vi "Modbus Close.vi"(8 "error in (no error)":errorcluster, 11 "VISA resource in":refnum<visa-resource-name>) -> (0 "error out":errorcluster)   [LabVIEW 2023, in "Voegtlin_NI_SMART_Modbus_Drivers.lvlib"]
doc: "Schlisst die Modbus-Verbingung und gibt den entsprechenden COM-Port wieder frei."
uses:
  Voegtlin_NI_SMART_Modbus_Drivers.lvlib
  Low Level Driver/Enums/Modbus Comm.ctl
panel:
  # "Input Data"
  # "Output Data"
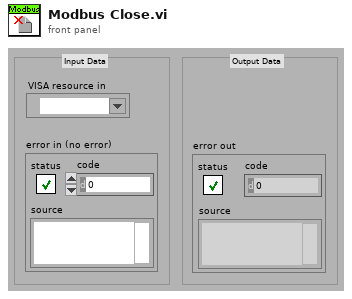
[diagram p1: front panel]
types:
  T1 = typedef "Voegtlin_NI_SMART_Modbus_Drivers.lvlib/Modbus Comm.ctl" = enum16{"Init", "Read", "Write", "Exit"}
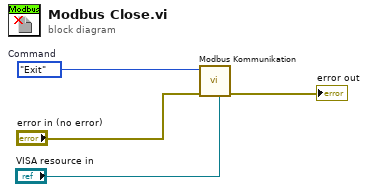
[diagram p0: block diagram]
diagram:
  w2 = Modbus_Comm."Exit"  # Command
  n1 = call "Modbus Kommunikation.vi"("VISA resource in"="VISA resource in", "error in (no error)"="error in (no error)", "Command"=w2) -> ("error out"=→"error out":errorcluster)  [unwired: 6 in, 2 out]
